vi "closeFile.vi"(8 "error in (no error)":errorcluster, 10 "Save? (F)":bool, 11 "Refnum Cluster In":T1) -> (0 "error out":errorcluster)   [LabVIEW 2012]
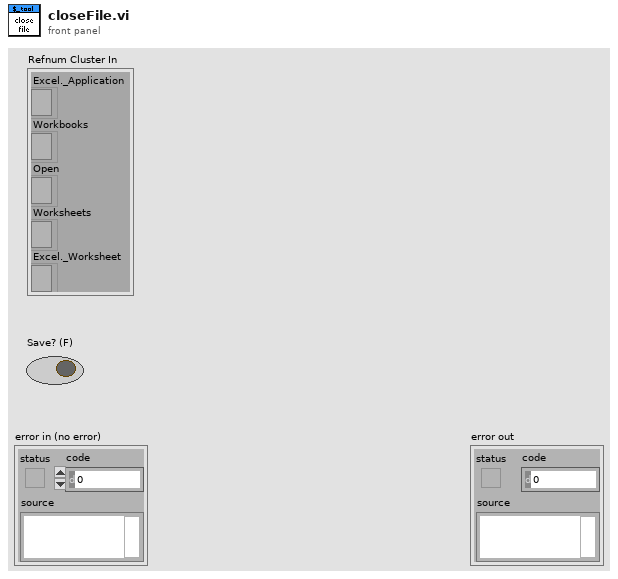
[diagram p1: front panel]
types:
  T1 = cluster{"Excel._Application":refnum<k7>, "Workbooks":refnum<k7>, "Open":refnum<k7>, "Worksheets":refnum<k7>, "Excel._Worksheet":refnum<k7>}
  T2 = cluster{"Excel._Application":refnum<k7>, "Workbooks":refnum<k7>, "Open":refnum<k7>}
  T3 = cluster{"Excel._Application":refnum<k7>, "Workbooks":refnum<k7>}
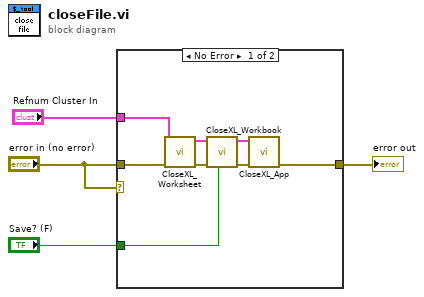
[diagram p0: block diagram]
diagram:
  n1 = case shown="No Error" "error in (no error)" {
    tunnel: "Save? (F)" -> [w11 _]
    tunnel: "error in (no error)" -> [w9 w13]
    tunnel: [w8 w13] -> w3
    tunnel: "Refnum Cluster In" -> [w5 _]
    frame No Error {
      n2 = call <userlib>:"CloseXL_Worksheet.vi"("error in (no error)"=w9, "Refnum Cluster In"=w5) -> ("error out"=w12:errorcluster, "Refnum Cluster Out"=w7:T2)  [unwired: 8 in]
      n3 = call <userlib>:"CloseXL_Workbook.vi"("Save? (F)"=w11, "error in (no error)"=w12, "Refnum Cluster In"=w7) -> ("error out"=w10:errorcluster, "Refnum Cluster Out"=w6:T3)  [unwired: 7 in]
      n4 = call <userlib>:"CloseXL_App.vi"("error in (no error)"=w10, "Refnum Cluster In"=w6) -> ("error out"=w8:errorcluster)  [unwired: 9 in]
    }
    frame Error {
    }
  }
  "error out" <- w3
